vi "Encrypt.vi"(8 "error in (no error)":errorcluster, 10 "Arguments":string[](array[string]), 11 "FFT in":refnum<class "FFT.lvclass">) -> (0 "error out":errorcluster, 2 "Encrypted Arguments":string[](array[string]), 3 "FFT out":refnum<class "FFT.lvclass">)   [LabVIEW 2019, in "TSC Event Logger.lvlib" / "FFT.lvclass"]
doc: "Encrypt the list of arguments that need to be \"obfuscated\" for the actual recording of the data. Will return an array of the encrypted arguments as outputs.\n\n<b>Code Developed By:</b>\nTechnology Service Corporation\nBloomington, IN 47403\nwww.tsc.com/atcs\n\nDeveloper:\nDaniel Coons"
uses:
  FFT.lvclass
  C:/Development/Open Source/tsc-event-logger/Encryption/Encryption.lvclass
  Encryption.lvclass/Encryption.ctl
  <vilib>/Analysis/2dsp.llb/Real FFT.vi
  Read Multiplier.vi
  Read SALT location.vi
  Read SALT.vi
  <vilib>/Analysis/NI_AALPro.lvlib
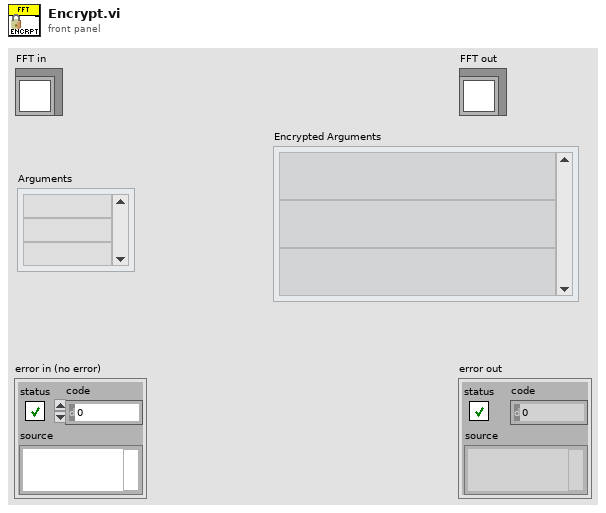
[diagram p1: front panel]
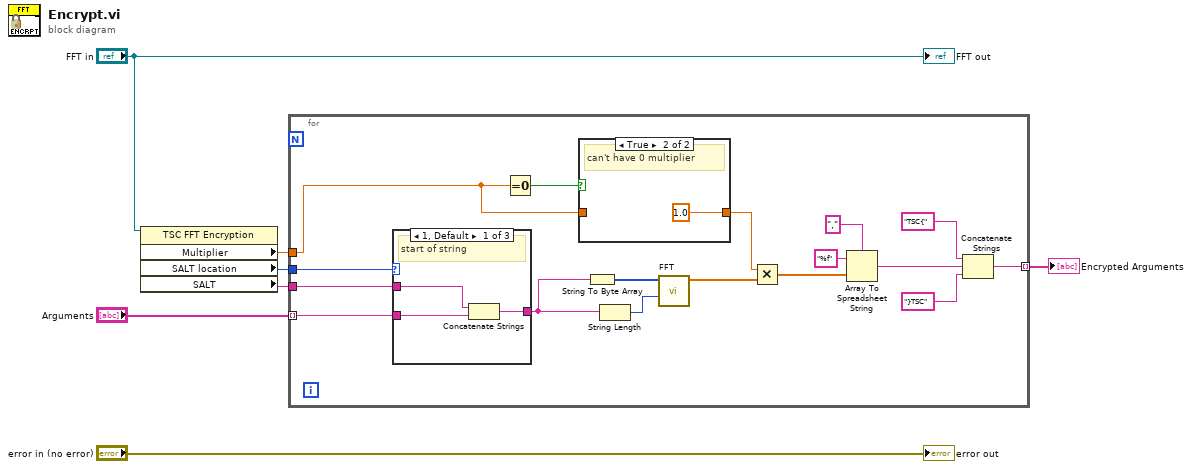
[diagram p0: block diagram]
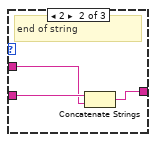
[diagram p3: hidden frame]
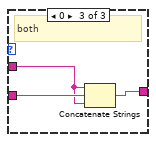
[diagram p4: hidden frame]
diagram:
  n1 = property class="TSC FFT Encryption"(reference="FFT in") -> ("Multiplier"=w1:dbl, "SALT location"=w2:u16, "SALT"=w5:string)  [unwired: 1 in, 2 out]
  n2 = for {
    tunnel: "Arguments" -> [w23] mode=indexing
    tunnel: [w22] -> w3 mode=indexing
    tunnel: w5 -> [w24]
    tunnel: w2 -> [w15]
    tunnel: w1 -> [w11]
    n3 = case shown="1, Default" w15 {
      tunnel: [w29 w32 w35] -> w16
      tunnel: w24 -> [w28 w30 w33]
      tunnel: w23 -> [w27 w31 w34]
      frame 1, Default {
        # "start of string"
        n4 = Concatenate Strings(w28, w27) -> (w29:string)
      }
      frame 2 {
        # "end of string"
        n5 = Concatenate Strings(w31, w30) -> (w32:string)
      }
      frame 0 {
        # "both"
        n6 = Concatenate Strings(w33, w34, w33) -> (w35:string)
      }
    }
    n7 = Equal To 0?(x=w11) -> (x = 0?=w12:bool)
    n8 = case shown="True" w12 {
      tunnel: w11 -> [w25 _]
      tunnel: [w25 1.0 ("Multiplier")] -> w10
      frame False {
        # "pass #"
      }
      frame True {
        # "can't have 0 multiplier"
      }
    }
    n9 = String To Byte Array(string=w16) -> (unsigned byte array=w17:u8[])
    n10 = String Length(string=w16) -> (length=w18:i32)
    n11 = call-poly <vilib>:"FFT.vi"("FFT size"=w18, "X"=w17) -> ("FFT {X}"=w19:cdb[])  [unwired: 8 in, 1 out]
    n12 = Multiply(x=w10, y=w19) -> (x*y=w14:cdb[])
    n13 = Array To Spreadsheet String(delimiter (Tab)=",", array=w14, 3:"%f" ("format string")) -> (spreadsheet string=w13:string)
    n14 = Concatenate Strings("TSC{" ("string"), w13, "}TSC" ("string")) -> (w22:string)
  }
  "Encrypted Arguments" <- w3
  "error out" <- "error in (no error)"
  "FFT out" <- "FFT in"
